vi "FPGA 64bit Timer.vi"() -> (0 "Current Time (us)":u64)   [LabVIEW 2015]
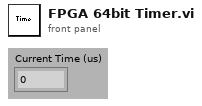
[diagram p1: front panel]
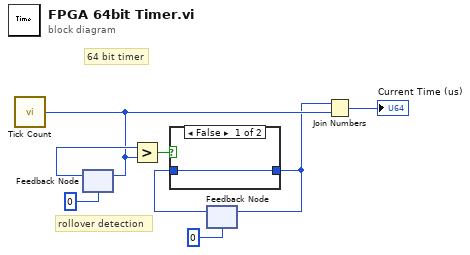
[diagram p0: block diagram]
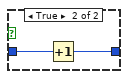
[diagram p2: hidden frame]
diagram:
  # "64 bit timer"
  # "rollover detection"
  n1 = call "Tick Count"() -> ("Tick Count(uSec)"=w7:u32)
  n2 = feedback-in #1(w7) -> ()
  n3 = feedback #1(u32 0 ("Tick Count(mSec)")) -> (w8:u32)
  n4 = Greater?(x=w8, y=w7) -> (0:w5:bool)
  n5 = feedback #2(u32 0 ("Tick Count(mSec)")) -> (w2:u32)
  n6 = case shown="False" w5 {
    tunnel: [w9 w11] -> w1
    tunnel: w2 -> [w9 w10]
    frame False {
    }
    frame True {
      n7 = Increment(x=w10) -> (x+1=w11:u32)
    }
  }
  n8 = feedback-in #2(w1) -> ()
  n9 = Join Numbers(hi=w1, lo=w7) -> ((hi.lo)=→"Current Time (us)":u64)
